vi "FeedbackSampleToWaveformArray.vi"(11 "FeedbackData":T1) -> (3 "WfArray":waveform(dbl)[](array[waveform]))   [LabVIEW 2019, in "ManualMode.lvlib"]
uses:
  ManualMode.lvlib
  Mark10 API/Cluster - FeedbackData.ctl
  <vilib>/Waveform/WDTOps.llb/WDT Append Waveforms DBL.vi
  <vilib>/Waveform/WDTOps.llb/WDT Number of Waveform Samples DBL.vi
  <vilib>/Waveform/WDTOps.llb/WDT Get Waveform Subset DBL.vi
  Mark10 API/Mark 10 TSTM-DC.lvlib
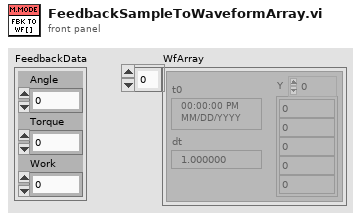
[diagram p1: front panel]
types:
  T1 = typedef "Mark 10 TSTM-DC.lvlib/Cluster - FeedbackData.ctl" = cluster{"Angle":dbl, "Torque":dbl, "Work":dbl}
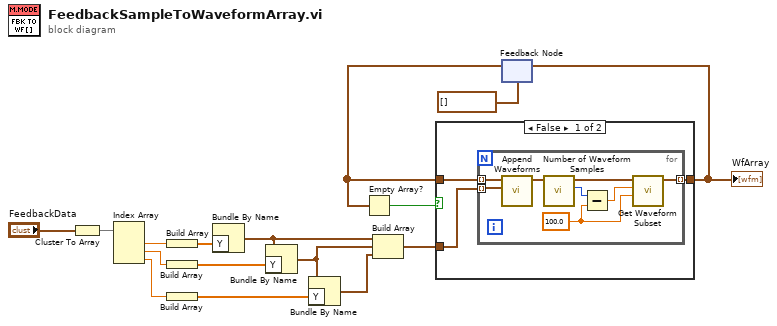
[diagram p0: block diagram]
diagram:
  n1 = Cluster To Array(cluster="FeedbackData") -> (array=w14:dbl[])
  n2 = Index Array(array=w14) -> (element #1=w13:dbl, element #2=w11:dbl, element #3=w10:dbl)  [unwired: 3 in]
  n3 = Build Array(w13) -> (w12:dbl[])
  n4 = Build Array(w11) -> (w9:dbl[])
  n5 = Build Array(w10) -> (w8:dbl[])
  n6 = Bundle By Name("Y"=w12) -> (w7:waveform(dbl))  [unwired: 1 in]
  n7 = Bundle By Name(cluster=w7, "Y"=w9) -> (w6:waveform(dbl))
  n8 = Bundle By Name(cluster=w6, "Y"=w8) -> (w5:waveform(dbl))
  n9 = Build Array(w7, w6, w5) -> (w4:waveform(dbl)[])
  n10 = feedback #1(waveform(dbl)[] []) -> (w3:waveform(dbl)[])
  n11 = Empty Array?(array=w3) -> (empty?=w2:bool)
  n12 = case shown="False" w2 {
    tunnel: w4 -> [w19 w28]
    tunnel: [w18 w28] -> w16
    tunnel: w3 -> [w17 _]
    frame False {
      n13 = for {
        tunnel: w17 -> [w27] mode=indexing
        tunnel: w19 -> [w26] mode=indexing
        tunnel: [w24] -> w18 mode=indexing
        w21 = 100.0 ("duration")
        n14 = call-poly <vilib>:"Append Waveforms.vi"("waveform B"=w26, "waveform A"=w27) -> ("waveform out"=w25:waveform(dbl))  [unwired: 8 in, 1 out]
        n15 = call-poly <vilib>:"Number of Waveform Samples.vi"("waveform in"=w25) -> ("number of samples"=w22:i32, "waveform out"=w23:waveform(dbl))  [unwired: 8 in, 1 out]
        n16 = Subtract(x=w22, y=w21) -> (x-y=w20:dbl)
        n17 = call-poly <vilib>:"Get Waveform Subset.vi"("duration"=w21, "start samples/time"=w20, "waveform in"=w23) -> ("waveform out"=w24:waveform(dbl))  [unwired: 3 in, 3 out]
      }
    }
    frame True {
    }
  }
  "WfArray" <- w16
  n18 = feedback-in #1(w16) -> ()
